vi "Create FileGlobal.vi"(0 "SequenceFile In":refnum<k7>, 11 "error in (no error)":errorcluster) -> (4 "SequenceFile Out":refnum<k7>, 15 "error out":errorcluster)   [LabVIEW 2021, in "Create Sequence.lvlib"]
uses:
  Create Sequence.lvlib
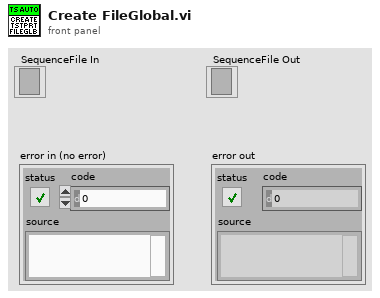
[diagram p1: front panel]
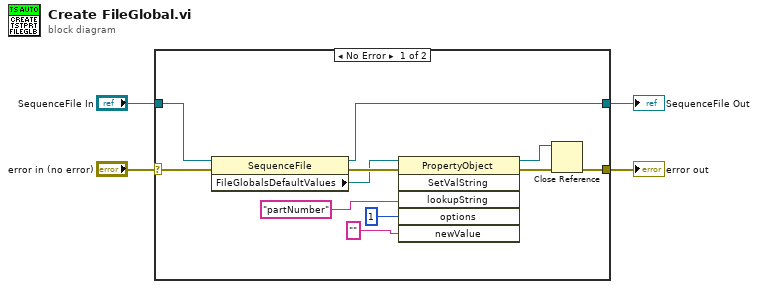
[diagram p0: block diagram]
diagram:
  n1 = case shown="No Error" "error in (no error)" {
    selector: "error in (no error)" -> [w5 w17]
    tunnel: [w9 w17] -> w4
    tunnel: [w7 w16] -> w3
    tunnel: "SequenceFile In" -> [w6 w16]
    frame No Error {
      n2 = property class="SequenceFile"(reference=w6, error in=w5) -> (reference out=w7:refnum<k7>, error out=w13:errorcluster, "FileGlobalsDefaultValues"=w12:refnum<k7>)
      n3 = invoke class="PropertyObject" method="SetValString"(reference=w12, error in=w13, "lookupString"="partNumber" ("Path"), "options"=1, "newValue"="") -> (reference out=w8:refnum<k7>, error out=w10:errorcluster)  [unwired: 1 in, 4 out]
      n4 = Close Reference(reference=w8, error in (no error)=w10) -> (error out=w9:errorcluster)
    }
    frame Error {
    }
  }
  "error out" <- w4
  "SequenceFile Out" <- w3
